vi "Write Vacuum StateQ.vi"(10 "Vacuum StateQ":refnum<queue>, 11 "Transfer Line in":refnum<class "Transfer Line.lvclass">) -> (3 "Transfer Line out":refnum<class "Transfer Line.lvclass">)   [LabVIEW 2015, in "cRIO-Carbondioxide.lvlib" / "CO2-Actor.lvlib" / "Transfer Line.lvclass"]
uses:
  Transfer Line.lvclass
  Controls/Vacuum State Cluster.ctl
  Controls/Vacuum State Enumerator.ctl
  Transfer Line.lvclass/Transfer Line.ctl
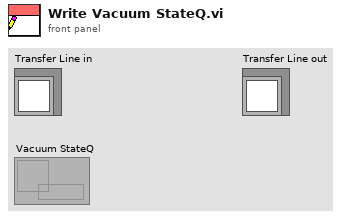
[diagram p1: front panel]
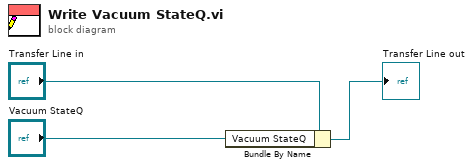
[diagram p0: block diagram]
diagram:
  n1 = Bundle By Name(cluster="Transfer Line in", "Vacuum StateQ"="Vacuum StateQ") -> (→"Transfer Line out":refnum<class "Transfer Line.lvclass">)
